vi "get_replyReceiver.vi"(0 "MoAgSy_Message":refnum<class "MoAgSy_Message.lvclass">, 5 "error in (no error)":errorcluster) -> (11 "GPG crypt":bool, 13 "sender ID":string, 14 "dup MoAgSy_Message":refnum<class "MoAgSy_Message.lvclass">, 16 "reply to":string, 17 "addressee":string, 19 "error out":errorcluster)   [LabVIEW 2009, in "MoAgSy.lvlib" / "MoAgSy_Message.lvclass"]
uses:
  MoAgSy_Message.lvclass
  MoAgSy_Message.lvclass/MoAgSy_Message.ctl
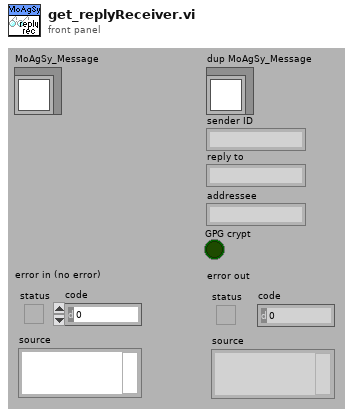
[diagram p1: front panel]
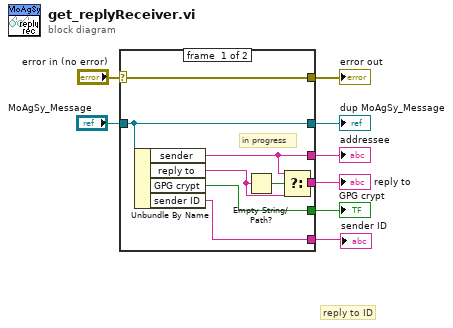
[diagram p0: block diagram]
diagram:
  # "reply to ID"
  n1 = case shown="No Error" "error in (no error)" {
    selector: "error in (no error)" -> [w16 w18]
    tunnel: [w16 w18] -> w7
    tunnel: [w15 w17] -> w5
    tunnel: "MoAgSy_Message" -> [w15 w17]
    tunnel: [w12 _] -> w4
    tunnel: [w11 _] -> w3
    tunnel: [w10 _] -> w2
    tunnel: [w9 _] -> w1
    frame #0 {
      # "in progress"
      n2 = Unbundle By Name(w15) -> ("sender"=w11:string, "reply to"=w13:string, "GPG crypt"=w10:bool, "sender ID"=w9:string)
      n3 = Empty String/Path?(string/path=w13) -> (empty?=w14:bool)
      n4 = Select(t=w11, s=w14, f=w13) -> (s? t:f=w12:string)
    }
    frame #1 {
    }
  }
  "error out" <- w7
  "dup MoAgSy_Message" <- w5
  "reply to" <- w4
  "addressee" <- w3
  "GPG crypt" <- w2
  "sender ID" <- w1
